vi "SelectImage.vi"(1 "Selected Slide":refnum<vi>, 2 "LUT":T1(array[cluster]), 3 "Desired Dimensions":cluster{"Width":i32, "Height":i32}={"Width"=100, "Height"=100}, 4 "Mouse Position":cluster{"X":i32, "Y":i32}) -> (5 "Offset":cluster{"X":i32, "Y":i32}, 6 "Name":string, 7 "slide":i32)   [LabVIEW 2012]
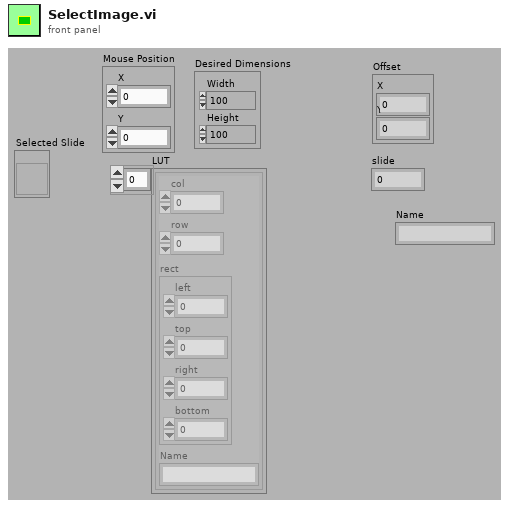
[diagram p1: front panel]
types:
  T1 = cluster{"col":i32, "row":i32, "rect":cluster{"left":i16, "top":i16, "right":i16, "bottom":i16}, "Name":string}[]
  T2 = cluster{"col":i32, "row":i32, "rect":cluster{"left":i16, "top":i16, "right":i16, "bottom":i16}, "Name":string}
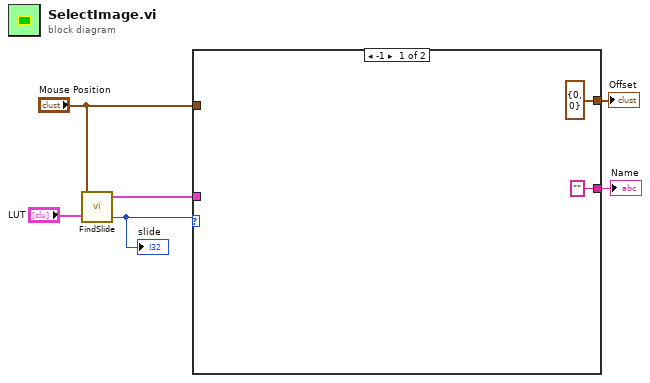
[diagram p0: block diagram]
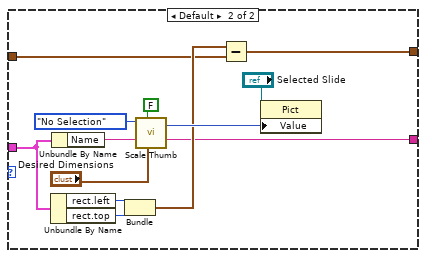
[diagram p2: hidden frame]
diagram:
  n1 = call "FindSlide.vi"("LUT"="LUT", "Mouse Position"="Mouse Position") -> ("slide"=w2:i32, "position"=w5:T2)  [unwired: 1 in]
  "slide" <- w2
  n2 = case shown="-1" w2 {
    tunnel: w5 -> [_ w15]
    tunnel: [cluster{i32, i32} {0, 0} w13] -> w4
    tunnel: "Mouse Position" -> [_ w12]
    tunnel: ["" ("Name") w9] -> w1
    frame -1 {
    }
    frame Default {
      n3 = Unbundle By Name(w15) -> ("rect.left"=w17:i16, "rect.top"=w16:i16)
      n4 = Unbundle By Name(w15) -> ("Name"=w9:string)
      n5 = Bundle("left"=w17, "top"=w16) -> (w14:cluster{"left":i16, "top":i16})  [unwired: 1 in]
      n6 = call "Scale Thumb.vi"("Desired Dimensions"="Desired Dimensions", "Full Size"=FALSE ("Show Labels"), "file"=w9, "Mod"=enum32{"No Selection", "Bounce", "Order"}."No Selection") -> ("new picture"=w18:picture)  [unwired: 2 in, 1 out]
      n7 = Subtract(x=w14, y=w12) -> (x-y=w13:cluster{i32, i32})
      n8 = property on="Property Node" class="Pict"(reference="Selected Slide", "Value"=w18) -> ()  [unwired: 1 in, 2 out]
    }
  }
  "Offset" <- w4
  "Name" <- w1
